vi "4.3.vi"() -> ()   [LabVIEW 2017]
panel:
  out "数值 3":dbl
  in  "x":dbl
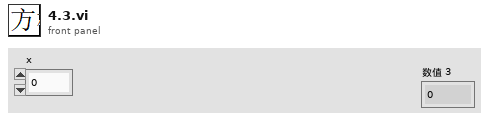
[diagram p1: front panel]
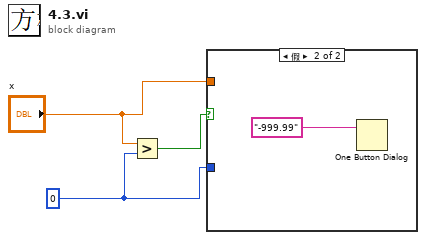
[diagram p0: block diagram]
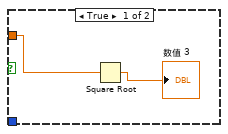
[diagram p2: hidden frame]
diagram:
  w1 = 0
  n1 = Greater?(x="x", y=w1) -> (0:w3:bool)
  n2 = case shown="假" w3 {
    tunnel: w1 -> [_ _]
    tunnel: "x" -> [w5 _]
    frame True {
      n3 = Square Root(x=w5) -> (sqrt(x)=→"数值 3":dbl)
    }
    frame False {
      n4 = One Button Dialog(message="-999.99") -> ()  [unwired: 1 in, 1 out]
    }
  }
